vi "oneDtext2array(str).vi"(11 "String":string="\\voltsPerGram.txt") -> (3 "text":string[](array[string]))   [LabVIEW 2017]
uses:
  <vilib>/Utility/file.llb/Read Delimited Spreadsheet (string).vi
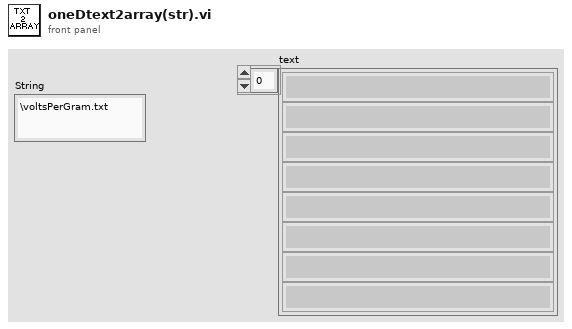
[diagram p1: front panel]
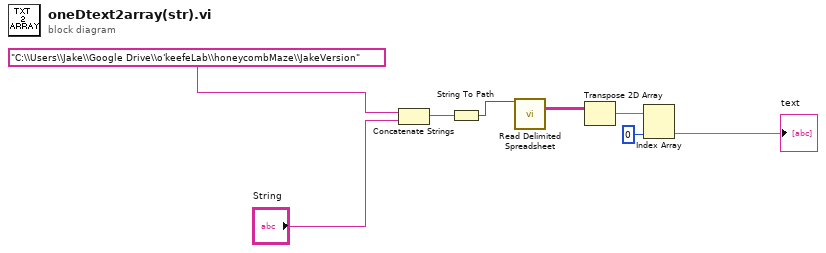
[diagram p0: block diagram]
diagram:
  n1 = Concatenate Strings("C:\\Users\\Jake\\Google Drive\\o'keefeLab\\honeycombMaze\\JakeVersion", "String") -> (w5:string)
  n2 = String To Path(string=w5) -> (path=w4:path)
  n3 = call-poly <vilib>:"Read Delimited Spreadsheet.vi"("file path (dialog if empty)"=w4) -> ("all rows"=w8:string[][])  [unwired: 9 in, 5 out]
  n4 = Transpose 2D Array(2D array=w8) -> (transposed array=w7:string[][])
  n5 = Index Array(array=w7, index (col)=0 ("disabled index (col)")) -> (element=→"text":string[])  [unwired: 1 in]
